vi "Fulfull (Value).vi"(8 "error in (no error)":errorcluster, 10 "Value":variant, 11 "Future in":refnum<class "Future.lvclass">) -> (0 "error out":errorcluster)   [LabVIEW 2017, in "Promise Future.lvlib" / "Future.lvclass"]
uses:
  Future.lvclass
  Future.lvclass/Future.ctl
  State/State.lvclass
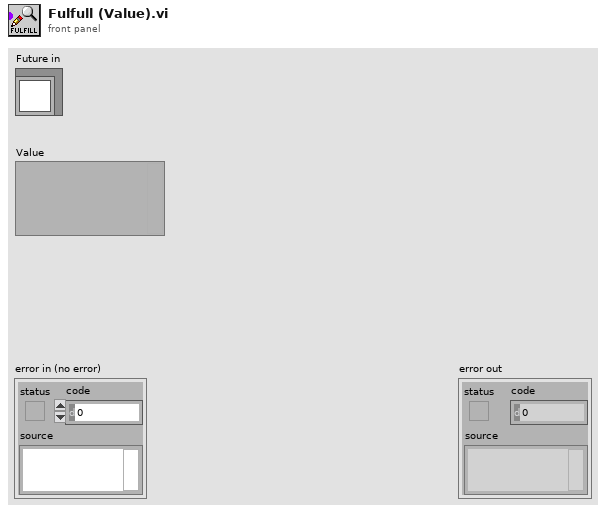
[diagram p1: front panel]
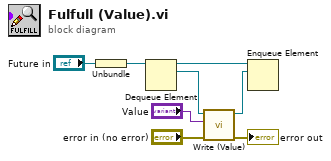
[diagram p0: block diagram]
diagram:
  n1 = Unbundle("Future in") -> (w8:refnum<queue>)
  n2 = Dequeue Element(queue=w8) -> (queue out=w7:refnum<queue>, element=w5:refnum<class "State.lvclass">)  [unwired: 2 in, 2 out]
  n3 = call "Write (Value).vi"("error in (no error)"="error in (no error)", "Value"="Value", "State in"=w5) -> ("error out"=→"error out":errorcluster, "State out"=w3:refnum<class "State.lvclass">)  [unwired: 7 in]
  n4 = Enqueue Element(queue=w7, element=w3) -> ()  [unwired: 2 in, 3 out]
